vi "Shorten Wheel Type String.vi"(11 "wheel type":string) -> (3 "short wheel type":string)   [LabVIEW 2017, in "NI_Robotics_Configure Steering Frame.lvlib"]
uses:
  <vilib>/robotics/Dialog/Configure Steering Frame/NI_Robotics_Configure Steering Frame.lvlib
panel:
  out "found?":bool
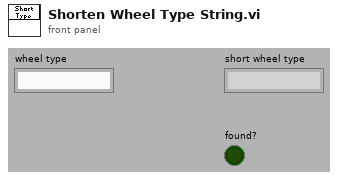
[diagram p1: front panel]
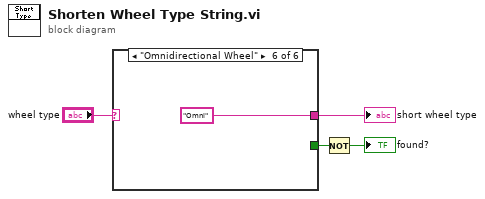
[diagram p0: block diagram]
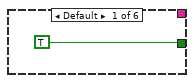
[diagram p2: hidden frame]
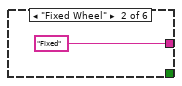
[diagram p3: hidden frame]
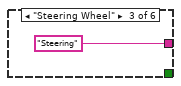
[diagram p4: hidden frame]
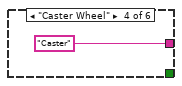
[diagram p5: hidden frame]
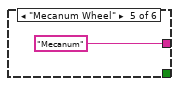
[diagram p6: hidden frame]
diagram:
  n1 = case shown="\"Omnidirectional Wheel\"" "wheel type" {
    tunnel: [TRUE _ _ _ _ _] -> w2
    tunnel: [_ "Fixed" "Steering" "Caster" "Mecanum" "Omni"] -> w1
    frame Default {
    }
    frame "Fixed Wheel" {
    }
    frame "Steering Wheel" {
    }
    frame "Caster Wheel" {
    }
    frame "Mecanum Wheel" {
    }
    frame "Omnidirectional Wheel" {
    }
  }
  "short wheel type" <- w1
  n2 = Not(x=w2) -> (.not. x?=→"found?":bool)
